vi "ConsolidateTasks.vi"(10 "Tasks":refnum<k21>[](array[refnum]), 11 "Task Name":string="All Channels Task") -> (1 "Cancelled?":bool, 2 "Task Out":refnum<k21>)   [LabVIEW 2013]
uses:
  Popups/Progress Bar Actions.ctl
  <vilib>/Utility/error.llb/DialogType.ctl
  Instance           1 27Saved   GenerateTestAllTask .vi
  <vilib>/DAQmx/create/channels.llb/DAQmx Create Channel (AI-Voltage-Basic).vi
  <vilib>/DAQmx/create/channels.llb/DAQmx Create Channel (AI-Strain-Strain Gage).vi
  <vilib>/DAQmx/create/channels.llb/DAQmx Create Channel (AI-Position-LVDT).vi
  <vilib>/DAQmx/create/channels.llb/DAQmx Create Channel (AI-Position-RVDT).vi
  <resource>/objmgr/daqmx.rc
panel:
  out "error out":errorcluster
  in  "error in (no error)":errorcluster
  out "AI.MeasType":i32(ring)=10300 items=["Voltage"=10322, "Current"=10134, "More:Voltage:Custom with Excitation"=10323, "Frequency"=10181, "Resistance"=10278, "Temperature:Thermocouple"=10303, "Temperature:Thermistor"=10302, "Temperature:RTD"=10301, "Temperature:Built-in Sensor"=10311, "Strain Gage"=10300, "Position:LVDT"=10352, "Position:RVDT"=10353, "Accelerometer"=10356, "Sound Pressure:Microphone"=10354, "TEDS Sensor"=12531]
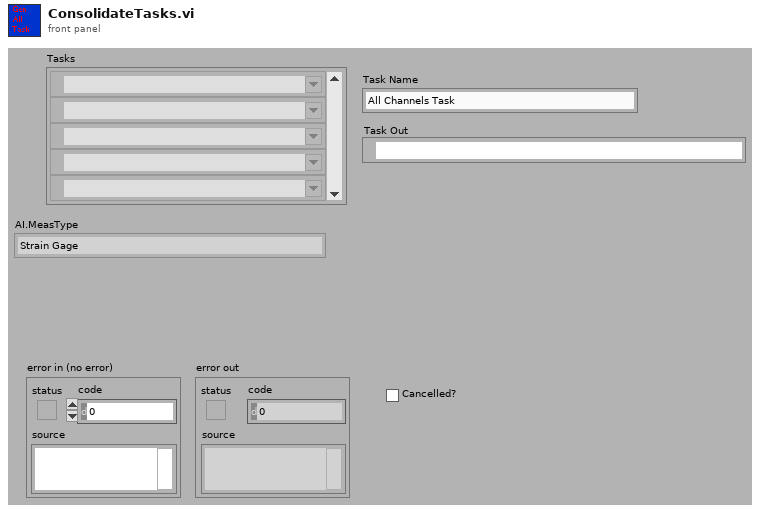
[diagram p1: front panel]
types:
  T1 = typedef "Progress Bar Actions.ctl" = enum16{"Get", "Set", "Exit", "Init"}
  T2 = cluster{"gage factor":dbl, "nominal gage resistance":dbl, "poisson ratio":dbl}
  T3 = cluster{"strain configuration":i32, "lead wire resistance":dbl, "initial bridge voltage":dbl, "voltage excitation source":i32, "voltage excitation value":dbl}
  T4 = typedef "DialogType.ctl" = u16
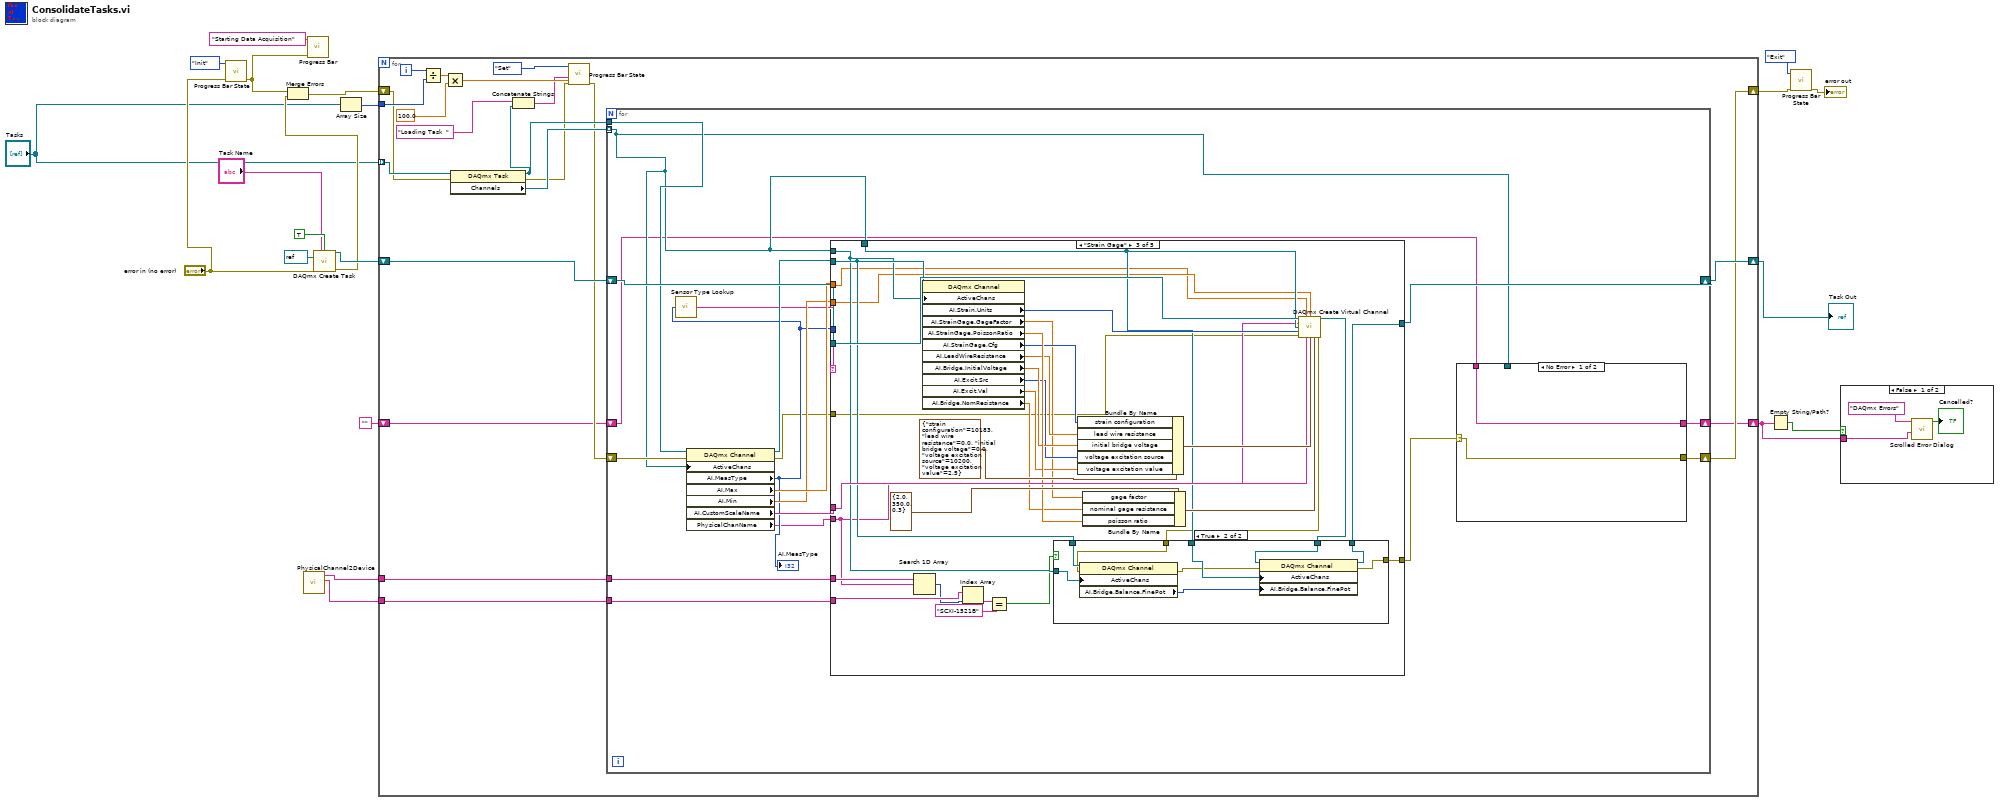
[diagram p0: block diagram]
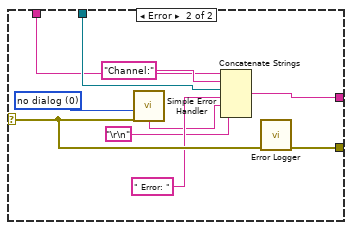
[diagram p3: hidden frame]
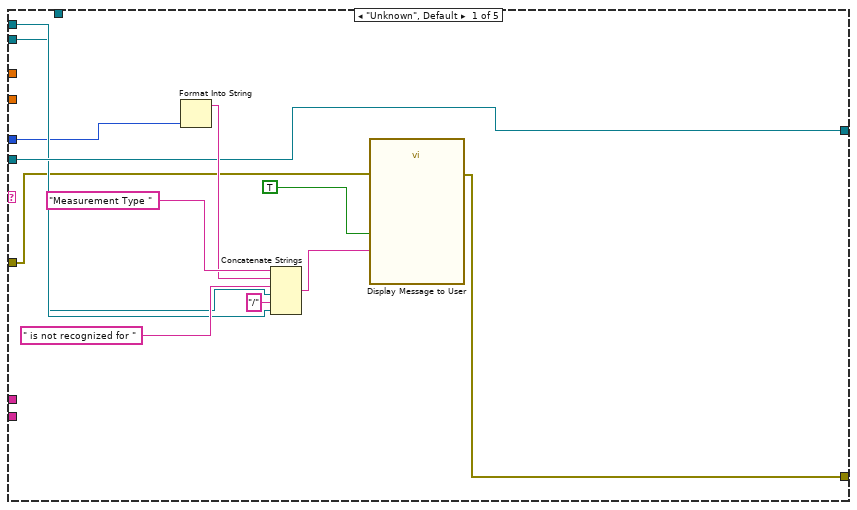
[diagram p4: hidden frame]
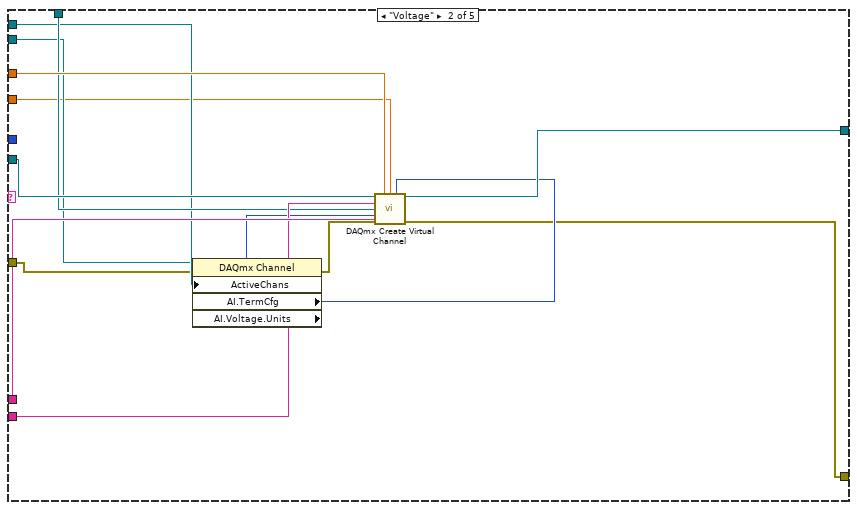
[diagram p5: hidden frame]
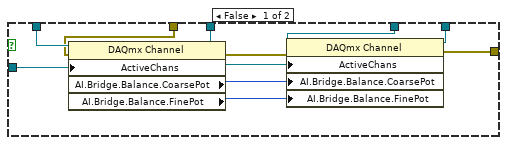
[diagram p6: hidden frame]
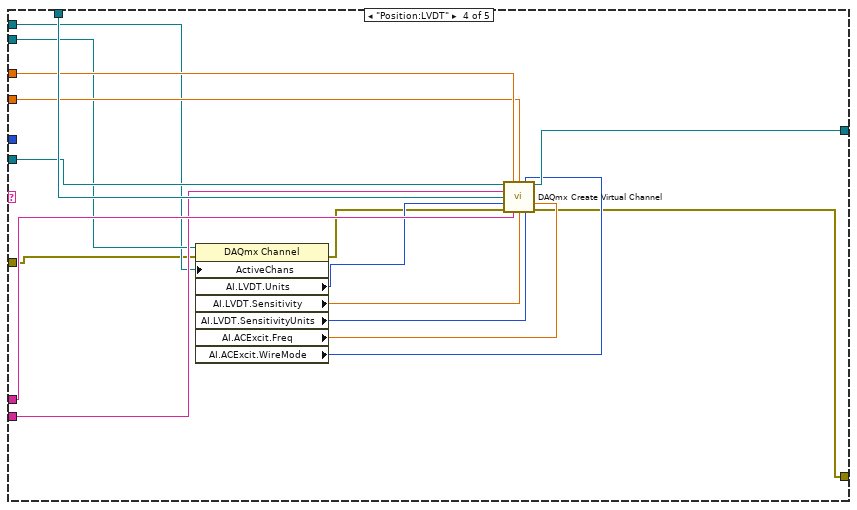
[diagram p7: hidden frame]
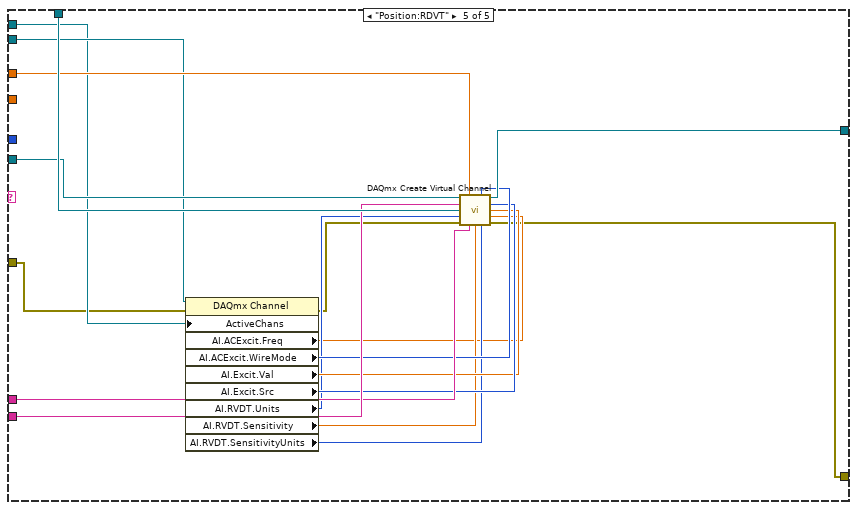
[diagram p8: hidden frame]
diagram:
  n1 = call "Progress Bar State.vi"("error in (no error)"="error in (no error)", "Progress Actions"=Progress_Bar_Actions."Init") -> ("error out"=w9:errorcluster)  [unwired: 2 in, 7 out]
  n2 = call "PhysicalChannel2Device.vi"() -> ("Associated Device"=w15:string[], "Physical Channels"=w16:tag[])  [unwired: 10 out]
  n3 = call "Progress Bar.vi"("error in (no error)"=w9, "Label In"="Starting Data Acquisition") -> ()  [unwired: 10 out]
  n4 = call <vilib>:"DAQmx Create Task.vi"("new task name"="Task Name", "auto cleanup"=TRUE, "task to copy"=refnum<k21> refnum, "error in"="error in (no error)") -> ("task out"=w19:refnum<k21>, "error out"=w6:errorcluster)  [unwired: 1 in, 9 out]
  n5 = Merge Errors(w9, w6) -> (w7:errorcluster)
  n6 = Array Size(array="Tasks") -> (size(s)=w12:i32)
  n7 = for {
    tunnel: "Tasks" -> [w42] mode=indexing
    shift-right: [w39] -> w18
    shift-left: w19 -> [w40]
    tunnel: w16 -> [w38]
    tunnel: w15 -> [w37]
    tunnel: w12 -> [w34]
    shift-right: [w24] -> w11
    shift-left: w7 -> [w27]
    shift-right: [w23] -> w2
    shift-left: "" -> [w22]
    i -> [w35]
    n8 = Divide(x=w35, y=w34) -> (x/y=w33:dbl)
    n9 = Multiply(x=w33, y=100.0) -> (x*y=w31:dbl)
    n10 = property class="DAQmx Task"(reference=w42, error in=w27) -> (reference out=w29:refnum<k21>, error out=w26:errorcluster, "Channels"=w41:refnum<k21>[])
    n11 = Concatenate Strings("Loading Task  " ("string"), w29) -> (w28:string)
    n12 = call "Progress Bar State.vi"("error in (no error)"=w26, "String In"=w28, "Progress In"=w31, "Progress Actions"=Progress_Bar_Actions."Set") -> ("error out"=w25:errorcluster)  [unwired: 7 out]
    n13 = for {
      tunnel: w41 -> [w47] mode=indexing
      tunnel: w29 -> [w59]
      shift-right: [w60] -> w39
      shift-left: w40 -> [w61]
      tunnel: w38 -> [w58]
      tunnel: w37 -> [w57]
      shift-right: [w45] -> w24
      shift-left: w25 -> [w56]
      shift-right: [w44] -> w23
      shift-left: w22 -> [w43]
      n14 = property class="DAQmx Channel"(reference=w59, error in=w56, "ActiveChans"=w47) -> (reference out=w53:refnum<k21>, error out=w48:errorcluster, "AI.MeasType"=w51:i32, "AI.Max"=w55:dbl, "AI.Min"=w52:dbl, "AI.CustomScaleName"=w54:tag, "PhysicalChanName"=w49:tag)
      "AI.MeasType" <- w51
      n15 = call "Sensor Type Lookup.vi"("AI.MeasType"=w51) -> ("String Rep"=w50:string)
      n16 = case shown="\"Strain Gage\"" w50 {
        tunnel: w61 -> [w80 w99 w131 w158 w183]
        tunnel: [w80 w98 w113 w163 w180] -> w60
        tunnel: w55 -> [_ w97 w100 w166 w184]
        tunnel: w54 -> [_ w96 w126 w165 w181]
        tunnel: w49 -> [_ w95 w109 w164 w182]
        tunnel: w47 -> [_ w94 w114 w167 w185]
        tunnel: w47 -> [w78 w93 w115 w154 w171]
        tunnel: w53 -> [w77 w90 w116 w156 w173]
        tunnel: w52 -> [_ w89 w101 w157 _]
        tunnel: w51 -> [w76 _ _ _ _]
        tunnel: w58 -> [_ _ w111 _ _]
        tunnel: w57 -> [_ _ w110 _ _]
        tunnel: w48 -> [w75 w88 w104 w153 w170]
        tunnel: [w74 w86 w102 w151 w168] -> w46
        frame "Unknown", Default {
          n17 = Format Into String(w76) -> (resulting string=w84:string)  [unwired: 3 in, 1 out]
          n18 = Concatenate Strings("Measurement Type " ("string"), w84, " is not recognized for " ("string"), w77, "/" ("string"), w78) -> (w82:string)
          n19 = call "Display Message to User"("error in (no error)"=w75, "Enable"=TRUE, "Message"=w82) -> ("error out"=w74:errorcluster)  [unwired: 8 out]
        }
        frame "Voltage" {
          n20 = property class="DAQmx Channel"(reference=w90, error in=w88, "ActiveChans"=w93) -> (error out=w87:errorcluster, "AI.TermCfg"=w92:i32, "AI.Voltage.Units"=w91:i32)  [unwired: 1 out]
          n21 = call-poly <vilib>:"DAQmx Create Virtual Channel.vi"("task in"=w99, "maximum value"=w97, "minimum value"=w89, "input terminal configuration"=w92, "physical channels"=w95, "name to assign"=w94, "units"=w91, "error in"=w87, "custom scale name"=w96) -> ("task out"=w98:refnum<k21>, "error out"=w86:errorcluster)  [unwired: 5 out]
        }
        frame "Strain Gage" {
          n22 = Search 1D Array(1D array=w111, element=w109) -> (index of element=w108:i32)  [unwired: 1 out]
          n23 = property class="DAQmx Channel"(reference=w116, "ActiveChans"=w115) -> ("AI.Strain.Units"=w119:i32, "AI.StrainGage.GageFactor"=w118:dbl, "AI.StrainGage.PoissonRatio"=w125:dbl, "AI.StrainGage.Cfg"=w124:i32, "AI.LeadWireResistance"=w123:dbl, "AI.Bridge.InitialVoltage"=w122:dbl, "AI.Excit.Src"=w121:i32, "AI.Excit.Val"=w120:dbl, "AI.Bridge.NomResistance"=w117:dbl)  [unwired: 1 in, 2 out]
          n24 = Index Array(array=w110, index=w108) -> (element=w107:string)
          n25 = Equal?(x=w107, y="SCXI-1521B") -> (x = y?=w105:bool)
          n26 = Bundle By Name(cluster=T3 {"strain configuration"=10183, "lead wire resistance"=0.0, "initial bridge voltage"=0.0, "voltage excitation source"=10200, "voltage excitation value"=2.5} ("bridge information"), "strain configuration"=w124, "lead wire resistance"=w123, "initial bridge voltage"=w122, "voltage excitation source"=w121, "voltage excitation value"=w120) -> (w129:T3)
          n27 = Bundle By Name(cluster=T2 {"gage factor"=2.0, "nominal gage resistance"=350.0, "poisson ratio"=0.3} ("strain gage information"), "gage factor"=w118, "nominal gage resistance"=w117, "poisson ratio"=w125) -> (w127:T2)
          n28 = call-poly <vilib>:"DAQmx Create Virtual Channel.vi"("task in"=w131, "maximum value"=w100, "minimum value"=w101, "physical channels"=w109, "name to assign"=w114, "units"=w119, "error in"=w104, "custom scale name"=w126, "bridge information"=w129, "strain gage information"=w127) -> ("task out"=w112:refnum<k21>, "error out"=w103:errorcluster)  [unwired: 1 in, 3 out]
          n29 = case shown="True" w105 {
            tunnel: w116 -> [w141 w145]
            tunnel: w115 -> [w140 w146]
            tunnel: w114 -> [w139 w149]
            tunnel: w112 -> [w137 w148]
            tunnel: [w136 w147] -> w113
            tunnel: w103 -> [w134 w144]
            tunnel: [w132 w142] -> w102
            frame False {
              n30 = property class="DAQmx Channel"(reference=w141, error in=w134, "ActiveChans"=w140) -> (error out=w133:errorcluster, "AI.Bridge.Balance.CoarsePot"=w138:i32, "AI.Bridge.Balance.FinePot"=w135:i32)  [unwired: 1 out]
              n31 = property class="DAQmx Channel"(reference=w137, error in=w133, "ActiveChans"=w139, "AI.Bridge.Balance.CoarsePot"=w138, "AI.Bridge.Balance.FinePot"=w135) -> (reference out=w136:refnum<k21>, error out=w132:errorcluster)
            }
            frame True {
              n32 = property class="DAQmx Channel"(reference=w145, error in=w144, "ActiveChans"=w146) -> (error out=w143:errorcluster, "AI.Bridge.Balance.FinePot"=w150:i32)  [unwired: 1 out]
              n33 = property class="DAQmx Channel"(reference=w148, error in=w143, "ActiveChans"=w149, "AI.Bridge.Balance.FinePot"=w150) -> (reference out=w147:refnum<k21>, error out=w142:errorcluster)
            }
          }
        }
        frame "Position:LVDT" {
          n34 = property class="DAQmx Channel"(reference=w156, error in=w153, "ActiveChans"=w154) -> (error out=w152:errorcluster, "AI.LVDT.Units"=w155:i32, "AI.LVDT.Sensitivity"=w162:dbl, "AI.LVDT.SensitivityUnits"=w161:i32, "AI.ACExcit.Freq"=w160:dbl, "AI.ACExcit.WireMode"=w159:i32)  [unwired: 1 out]
          n35 = call-poly <vilib>:"DAQmx Create Virtual Channel.vi"("task in"=w158, "maximum value"=w166, "minimum value"=w157, "voltage excitation wire mode"=w159, "physical channels"=w164, "name to assign"=w167, "units"=w155, "voltage excitation frequency"=w160, "error in"=w152, "custom scale name"=w165, "sensitivity"=w162, "sensitivity units"=w161) -> ("task out"=w163:refnum<k21>, "error out"=w151:errorcluster)  [unwired: 2 in]
        }
        frame "Position:RDVT" {
          n36 = property class="DAQmx Channel"(reference=w173, error in=w170, "ActiveChans"=w171) -> (error out=w169:errorcluster, "AI.ACExcit.Freq"=w172:dbl, "AI.ACExcit.WireMode"=w179:i32, "AI.Excit.Val"=w177:dbl, "AI.Excit.Src"=w178:i32, "AI.RVDT.Units"=w176:i32, "AI.RVDT.Sensitivity"=w175:dbl, "AI.RVDT.SensitivityUnits"=w174:i32)  [unwired: 1 out]
          n37 = call-poly <vilib>:"DAQmx Create Virtual Channel.vi"("task in"=w183, "maximum value"=w184, "voltage excitation wire mode"=w179, "physical channels"=w182, "voltage excitation source"=w178, "name to assign"=w185, "voltage excitation value"=w177, "units"=w176, "voltage excitation frequency"=w172, "error in"=w169, "custom scale name"=w181, "sensitivity"=w175, "sensitivity units"=w174) -> ("task out"=w180:refnum<k21>, "error out"=w168:errorcluster)  [unwired: 1 in]
        }
      }
      n38 = case shown="No Error" w46 {
        selector: w46 -> [w62 w73]
        tunnel: w47 -> [_ w70]
        tunnel: [w62 w64] -> w45
        tunnel: [w63 w66] -> w44
        tunnel: w43 -> [w63 w65]
        frame No Error {
        }
        frame Error {
          w72 = T4 0 items=["no dialog", "OK message", "continue or stop message", "OK message + warnings", "continue/stop + warnings"] ("type of dialog (OK msg:1)")
          n39 = call <vilib>:"Simple Error Handler.vi"("type of dialog (OK msg:1)"=w72, "error in (no error)"=w73) -> ("message"=w68:string)  [unwired: 7 out]
          n40 = Concatenate Strings(w65, "Channel:" ("string"), w70, " Error: " ("string"), w68, "\r\n") -> (w66:string)
          n41 = call "Error Logger.vi"("error in (no error)"=w73) -> ("error out"=w64:errorcluster)  [unwired: 10 in]
        }
      }
    }
  }
  "Task Out" <- w18
  n42 = Empty String/Path?(string/path=w2) -> (empty?=w3:bool)
  n43 = call "Progress Bar State.vi"("error in (no error)"=w11, "Progress Actions"=Progress_Bar_Actions."Exit") -> ("error out"=→"error out":errorcluster)  [unwired: 2 in, 7 out]
  n44 = case shown="False" w3 {
    tunnel: w2 -> [w187 _]
    frame False {
      n45 = call "Scrolled Error Dialog.vi"("Channels"=w187, "Title"="DAQmx Errors") -> ("Cancelled?"=→"Cancelled?":bool)  [unwired: 9 in]
    }
    frame True {
    }
  }
